vi "View.vi"(8 "error in (no error)":errorcluster, 11 "base view in":refnum<class "base view.lvclass">) -> (0 "error out":errorcluster, 3 "base view out":refnum<class "base view.lvclass">)   [LabVIEW 2022 SP3, in "base view.lvclass"]
uses:
  base view.lvclass
  Accessors/Read Event Registration Refnum.vi
  Accessors/Read View Refnum.vi
  base view.lvclass/base view.ctl
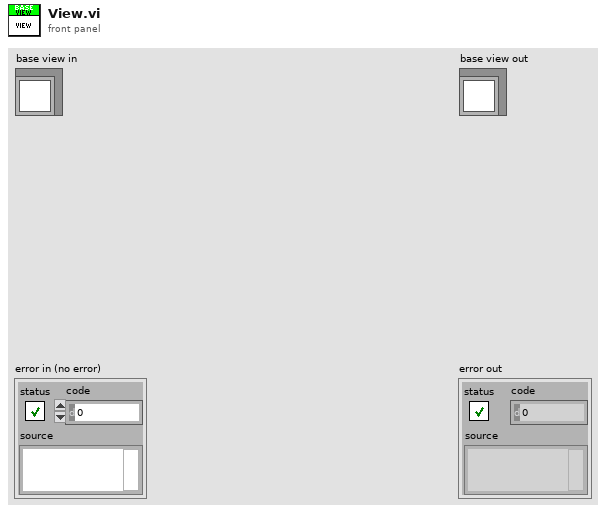
[diagram p1: front panel]
types:
  T1 = enum32{"Invalid", "Standard", "Closed", "Hidden", "Minimized", "Maximized"}
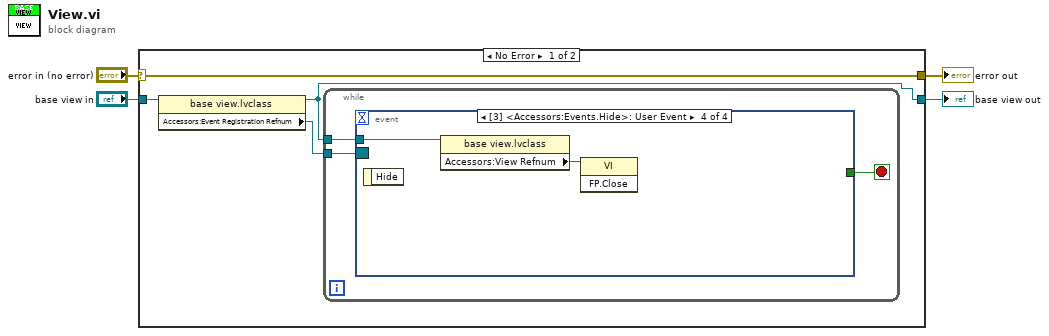
[diagram p0: block diagram]
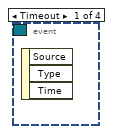
[diagram p2: hidden frame]
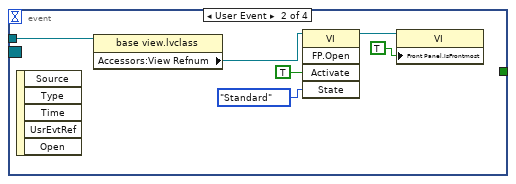
[diagram p3: hidden frame]
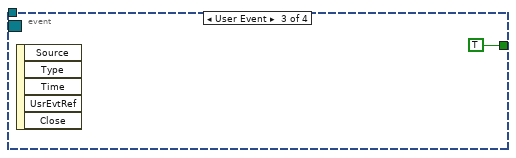
[diagram p4: hidden frame]
diagram:
  n1 = case shown="No Error" "error in (no error)" {
    selector: "error in (no error)" -> [w8 w22]
    tunnel: [w8 w22] -> w3
    tunnel: [w5 w21] -> w1
    tunnel: "base view in" -> [w7 w21]
    frame No Error {
      n2 = property class="base view.lvclass"(reference=w7) -> (reference out=w5:refnum<class "base view.lvclass">, "Accessors:Event Registration Refnum"=w6:refnum<event-registration>)  [unwired: 1 in, 1 out]
      n3 = while {
        tunnel: w6 -> [w11]
        tunnel: w5 -> [w9]
        stop <- w10 stop-if-true
        n4 = event shown="[3] <Accessors:Events.Hide>: User Event" {
          selector: w11 -> [_ _ _ _]
          dyn-events: _ -> [_ _ _ _]
          timeout: _ -> [_ _ _ _]
          tunnel: [_ _ TRUE _] -> w10
          tunnel: w9 -> [_ w17 _ w20]
          event Timeout {
            n5 = event-data() -> ()  [unwired: 1 in, 3 out]
          }
          event User Event {
            n6 = event-data() -> ()  [unwired: 1 in, 5 out]
            n7 = property class="base view.lvclass"(reference=w17) -> ("Accessors:View Refnum"=w16:refnum<vi>)  [unwired: 1 in, 2 out]
            n8 = invoke class="VI" method="FP.Open"(reference=w16, "Activate"=TRUE ("Activate?"), "State"=T1."Standard") -> (reference out=w13:refnum<vi>)  [unwired: 2 in, 4 out]
            n9 = property class="VI"(reference=w13, "Front Panel.IsFrontmost"=TRUE ("Front Panel Window:Is Frontmost")) -> ()  [unwired: 1 in, 2 out]
          }
          event User Event {
            n10 = event-data() -> ()  [unwired: 1 in, 5 out]
          }
          event User Event {
            n11 = event-data() -> ()  [unwired: 1 in, 1 out]
            n12 = property class="base view.lvclass"(reference=w20) -> ("Accessors:View Refnum"=w19:refnum<vi>)  [unwired: 1 in, 2 out]
            n13 = invoke class="VI" method="FP.Close"(reference=w19) -> ()  [unwired: 2 in, 3 out]
          }
        }
      }
    }
    frame Error {
    }
  }
  "error out" <- w3
  "base view out" <- w1
